vi "one - Server.vi"() -> ()   [LabVIEW 2015]
doc: "This is the TCP server VI that supports multiple connections from client VIs."
uses:
  TCP Multiple Connections/controls/TCP Multiple Connections State.ctl
  TCP Multiple Connections/controls/TCP Multiple Connections Data.ctl
  <vilib>/myRIO/Instrument Drivers/Onboard IO/AI/typedefs/AI Reference.ctl
  <vilib>/myRIO/Common/Instrument Driver Framework/Utilities/typedefs/myRIO Generic Hardware Reference.ctl
  <vilib>/myRIO/Common/Instrument Driver Framework/Utilities/typedefs/Hardware Version Enum.ctl
  <vilib>/myRIO/Common/Instrument Driver Framework/Utilities/typedefs/myRIO v1.0 Reference.ctl
  <vilib>/myRIO/Common/Instrument Driver Framework/Utilities/typedefs/Generic FPGA Reference.ctl
  <vilib>/myRIO/Common/Instrument Driver Framework/myRIO v1.0/AI/typedefs/AI Channels List.ctl
  <vilib>/myRIO/Common/Instrument Driver Framework/myRIO v1.0/AI/typedefs/AI Channels Enum.ctl
  <vilib>/myRIO/Common/Instrument Driver Framework/Utilities/typedefs/Analog Scaling Constants List.ctl
  <vilib>/myRIO/Common/Instrument Driver Framework/Utilities/typedefs/Analog Scaling Constants.ctl
  <vilib>/userdefined/High Color/nirio_resource_hc.ctl
  <vilib>/myRIO/Common/Instrument Driver Framework/Utilities/vis/Is FPGA Ref Available.vi
  <vilib>/myRIO/Common/Instrument Driver Framework/myRIO v1.0/AI/vis/myRIO v1.1 Open AI.vi
  <vilib>/myRIO/Instrument Drivers/Onboard IO/AI/vis/Read.vi
  <vilib>/myRIO/Common/Instrument Driver Framework/Utilities/vis/Validate Channels.vi
  <vilib>/myRIO/Common/Instrument Driver Framework/myRIO v1.0/AI/vis/myRIO v1.0 Reserve AI.vi
  <vilib>/myRIO/Common/Instrument Driver Framework/myRIO v1.0/AI/vis/myRIO v1.0 Build MUX Configuration AI.vi
  <vilib>/myRIO/Common/Instrument Driver Framework/myRIO v1.0/Resource Manager/vis/myRIO v1.0 Reserve Channel List.vi
  <vilib>/myRIO/Common/Instrument Driver Framework/myRIO v1.0/Resource Manager/vis/myRIO v1.0 Reserve Channel.vi
  <vilib>/myRIO/Common/Instrument Driver Framework/myRIO v1.0/Resource Manager/vis/myRIO v1.0 Unreserve Channel.vi
  <vilib>/myRIO/Common/Instrument Driver Framework/myRIO v1.0/Resource Manager/vis/myRIO v1.0 Build Mutex Name.vi
  <vilib>/Utility/VariantDataType/GetNumericInfo.vi
  <vilib>/Utility/error.llb/Error Cluster From Error Code.vi
  <vilib>/myRIO/Common/Instrument Driver Framework/myRIO v1.0/myRIO v1.1 Open.vi
  <vilib>/myRIO/Common/Instrument Driver Framework/myRIO v1.0/AI/vis/myRIO v1.0 Get Scaling Constants AI.vi
  <vilib>/myRIO/Common/Instrument Driver Framework/Utilities/vis/IO Manager.vi
  <vilib>/myRIO/Common/Instrument Driver Framework/Utilities/vis/Configuration Manager.vi
  <vilib>/myRIO/Common/Instrument Driver Framework/myRIO v1.0/myRIO v1.0 Close.vi
  <vilib>/myRIO/Common/Instrument Driver Framework/myRIO v1.0/AI/vis/myRIO v1.0 Read AI.vi
  <vilib>/myRIO/Express VI/Onboard IO/AI/AI Express VI.xnode
  <vilib>/myRIO/Instrument Drivers/Onboard IO/AI/vis/myRIO AI Open.xnode
  <vilib>/myRIO/Instrument Drivers/Onboard IO/AI/AI.lvlib
panel:
  out "String 6":string
  out "Waveform Chart 5":dbl(graph)
  out "String 5":string
  out "Waveform Chart 4":dbl(graph)
  out "String 4":string
  out "Waveform Chart 3":dbl(graph)
  in  "Stop":bool
  out "# of Connections":i32
  # "Overview: Demonstrates the use of the TCP functions to initialize a TCP server that can send data to multiple client VIs.\nInstructions:\n1. Run the VI.\n2. Open TCP Multiple Connections - Client 1.vi and follow the instructions on its front panel.\n3. Open TCP Multiple Connections - Client 2.vi and follow the instructions on its front panel.\n4. Click Stop to stop the VI."
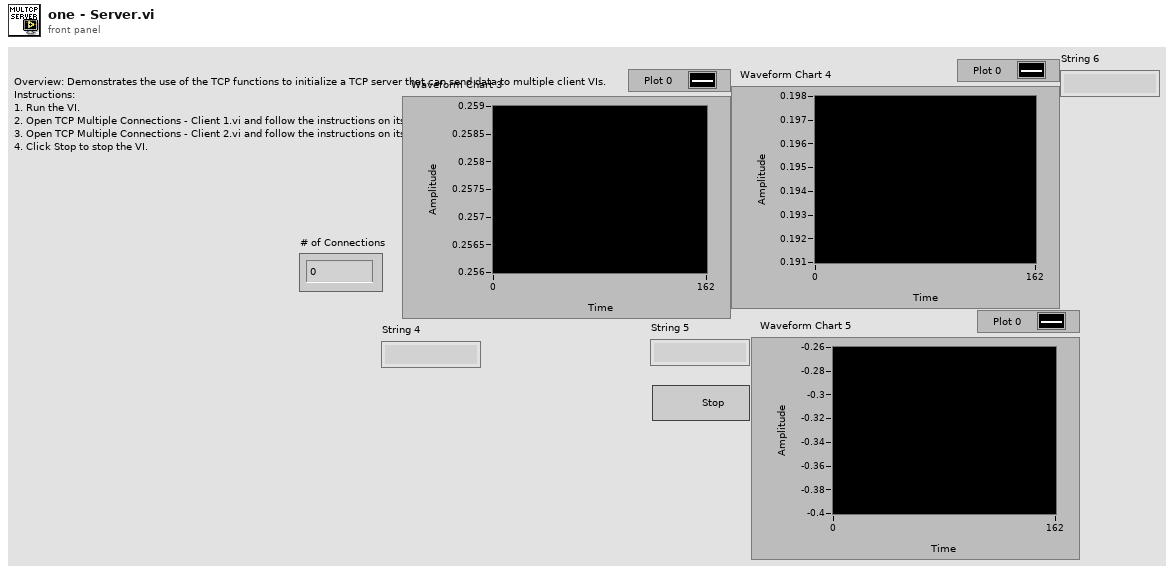
[diagram p1: front panel]
types:
  T1 = typedef "TCP Multiple Connections Data.ctl" = cluster{"Clients":refnum<k5>[], "Listener":refnum<k5>}
  T2 = typedef "TCP Multiple Connections State.ctl" = enum16{"Initialize", "Status Check", "Send Data", "Stop"}
  T3 = typedef "AI.lvlib/AI Reference.ctl" = cluster{"myRIO Reference":T4, "AI Channels List":T8, "AI Scaling Constants List":T10}
  T4 = typedef "myRIO Generic Hardware Reference.ctl" = cluster{"myRIO Model":T5, "myRIO Hardware Reference":T6}
  T5 = typedef "Hardware Version Enum.ctl" = enum16{"Unknown", "myRIO-1900", "myRIO-1950", "roboRIO"}
  T6 = typedef "myRIO v1.0 Reference.ctl" = cluster{"Generic FPGA Reference":T7, "Allow multiple opens":bool}
  T7 = typedef "Generic FPGA Reference.ctl" = refnum<k20>
  T8 = typedef "AI Channels List.ctl" = T9[]
  T9 = typedef "AI Channels Enum.ctl" = enum16{"Not Connected", "AudioIn/Left", "AudioIn/Right", "C/AI0", "C/AI1", "A/AI0", "A/AI1", "A/AI2", "A/AI3", "B/AI0", "B/AI1", "B/AI2", "B/AI3", "AI/AI0", "AI/AI1", "AI/AI2", "AI/AI3"}
  T10 = typedef "Analog Scaling Constants List.ctl" = T11[]
  T11 = typedef "Analog Scaling Constants.ctl" = cluster{"LSB Weight (Volts)":dbl, "Offset (Volts)":dbl, "Signed?":bool}
  T12 = typedef "nirio_resource_hc.ctl" = tag
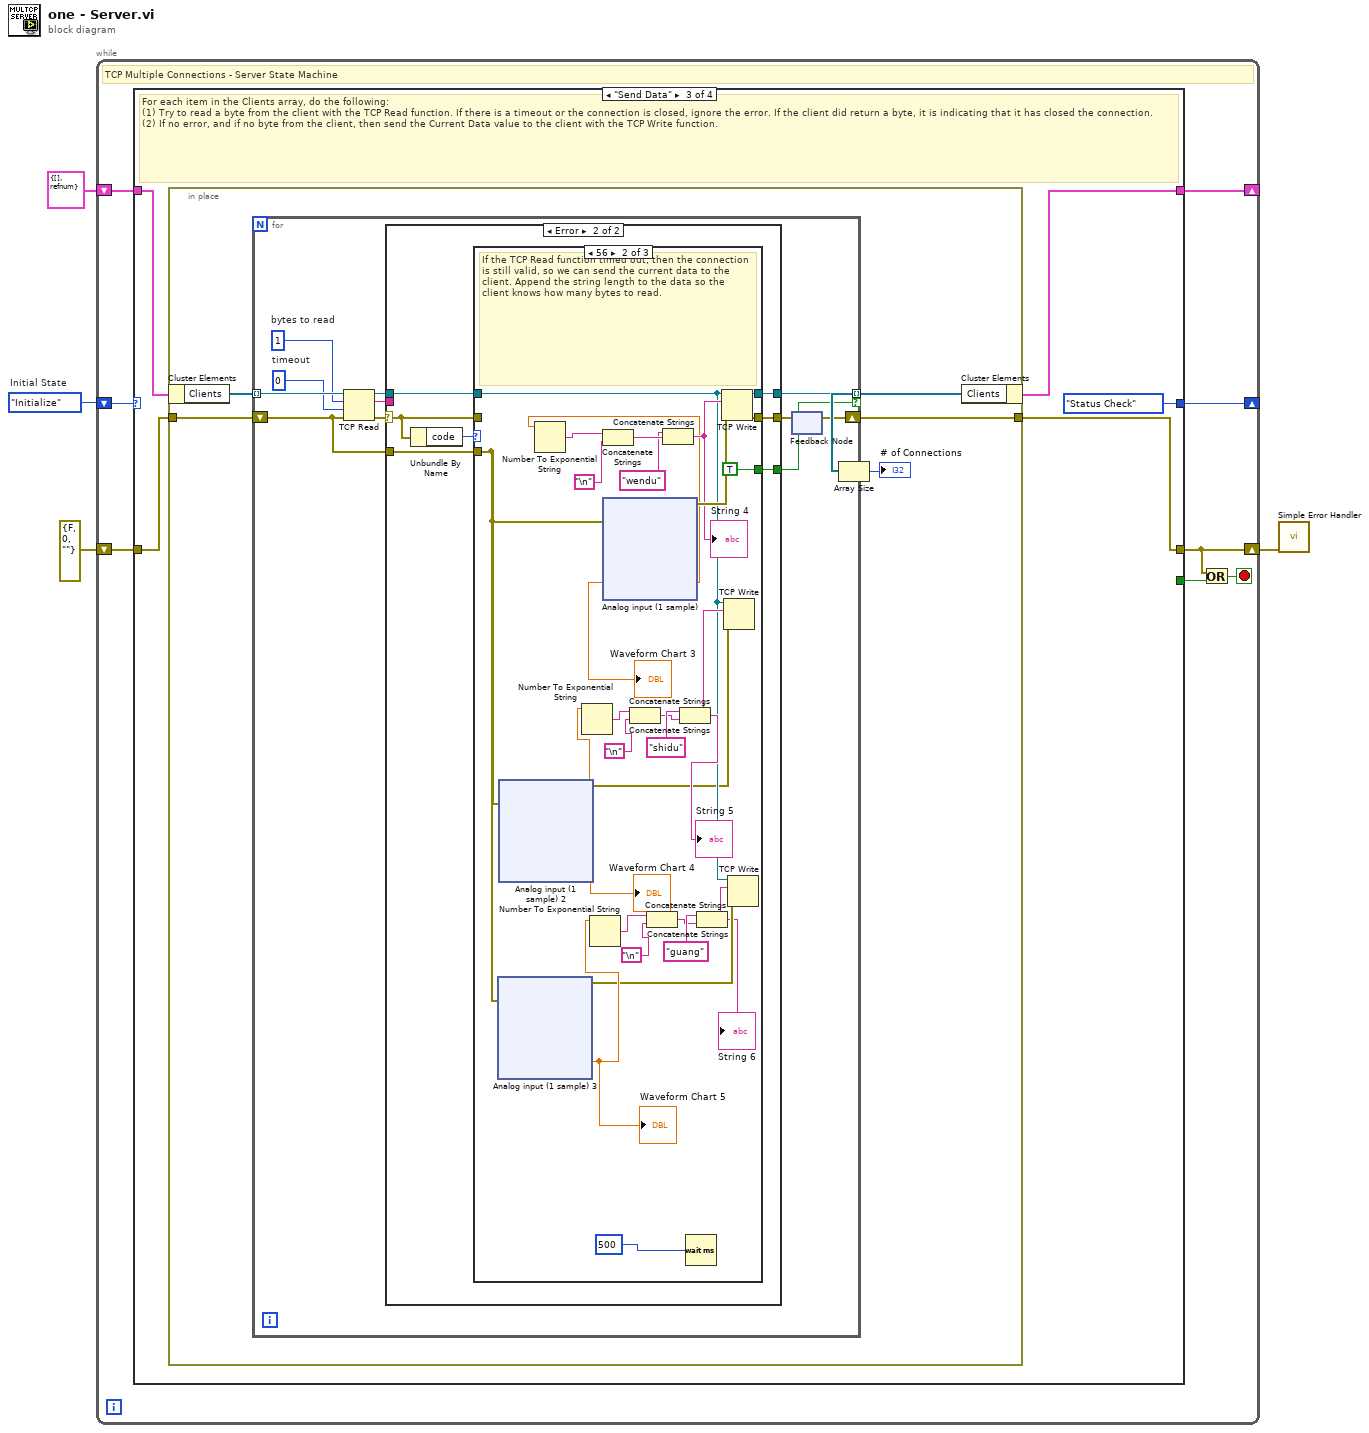
[diagram p0: block diagram]
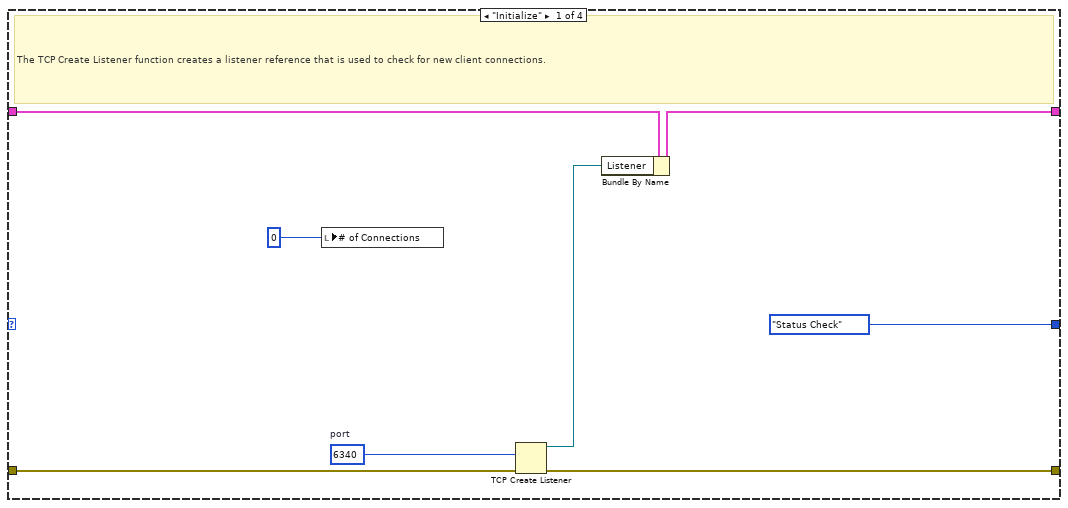
[diagram p2: hidden frame]
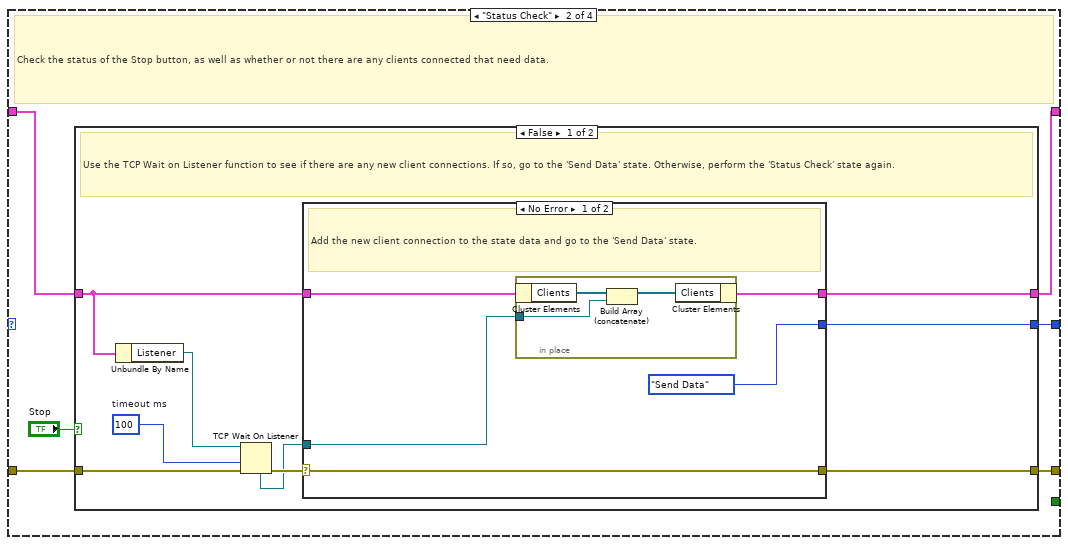
[diagram p3: hidden frame]
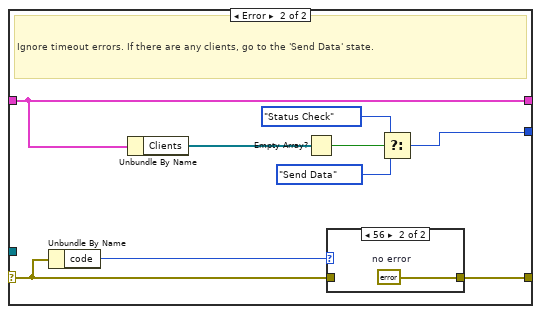
[diagram p4: hidden frame]
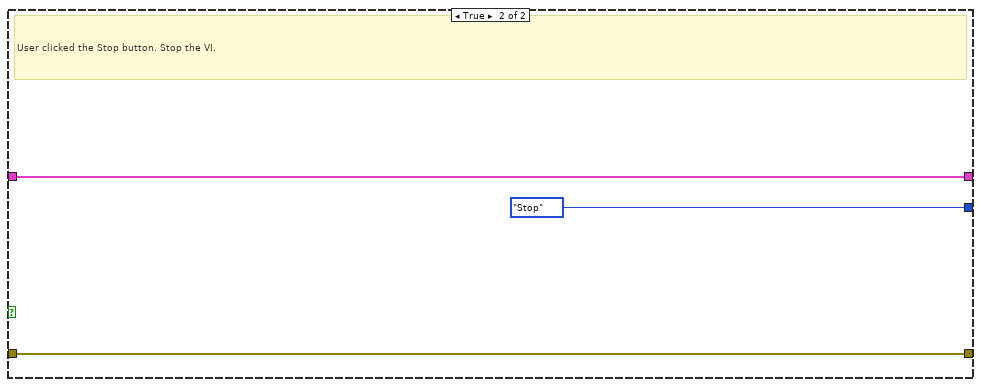
[diagram p6: hidden frame]
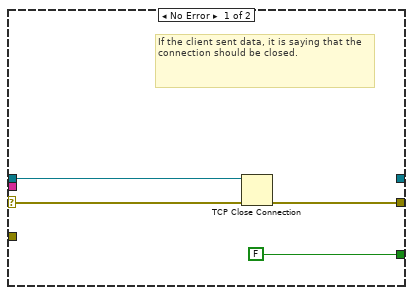
[diagram p7: hidden frame]
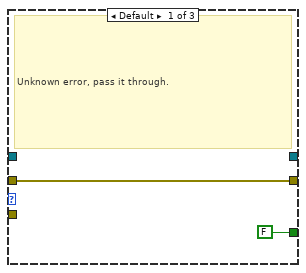
[diagram p8: hidden frame]
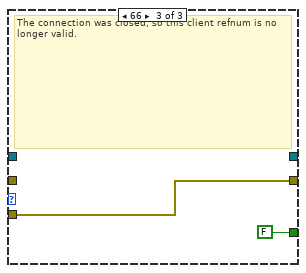
[diagram p9: hidden frame]
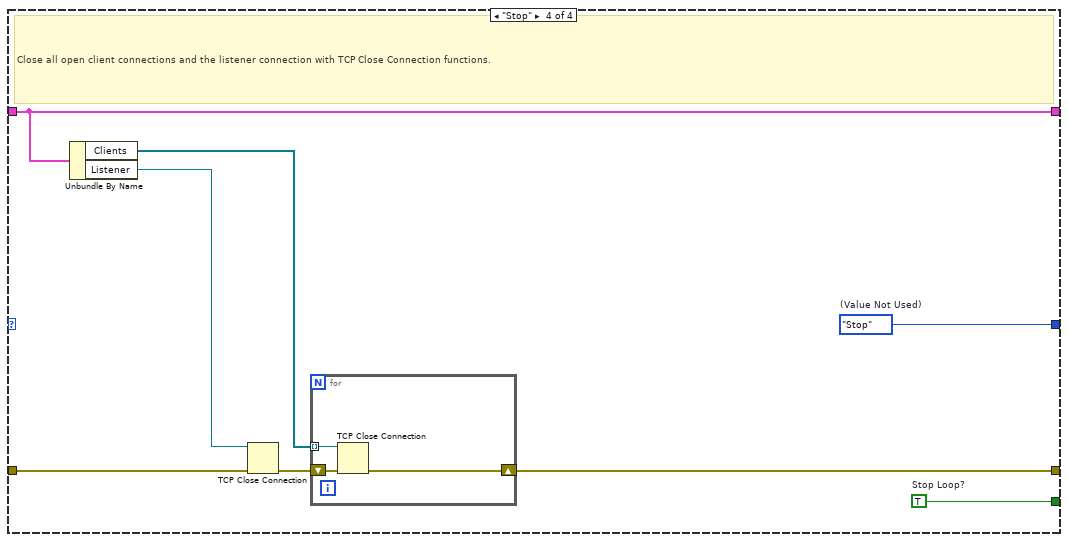
[diagram p10: hidden frame]
diagram:
  w4 = TCP_Multiple_Connections_State."Initialize"  # Initial State
  n1 = while {
    shift-right: [w11] -> _
    shift-left: w4 -> [w12]
    shift-right: [w9] -> _
    shift-left: T1 {"Clients"=[], "Listener"=refnum} ("Data") -> [w10]
    shift-right: [w5] -> w1
    shift-left: errorcluster {"status"=FALSE, "code"=0, "source"=""} ("error constant") -> [w8]
    stop <- w6 stop-if-true
    # "TCP Multiple Connections - Server State Machine"
    n2 = case shown="\"Send Data\"" w12 {
      tunnel: [TCP_Multiple_Connections_State."Status Check" ("States") w26 TCP_Multiple_Connections_State."Status Check" ("States") w232] -> w11
      tunnel: [_ _ _ w239] -> w7
      tunnel: w10 -> [w18 w22 w60 w238]
      tunnel: [w17 w21 w59 w238] -> w9
      tunnel: w8 -> [w20 w25 w62 w237]
      tunnel: [w19 w24 w61 w235] -> w5
      frame "Initialize" {
        w15 = u16 6340  # port
        # "The TCP Create Listener function creates a listener reference that is used to check for new client connections."
        n3 = local write "# of Connections"(0 ("Number of Client Connections")) -> ()
        n4 = TCP Create Listener(8:w20, 10:w15) -> (0:w19:errorcluster, 3:w16:refnum<k5>)  [unwired: 4 out]
        n5 = Bundle By Name(cluster=w18, "Listener"=w16) -> (w17:T1)
      }
      frame "Status Check" {
        # "Check the status of the Stop button, as well as whether or not there are any clients connected that need data."
        n6 = case shown="False" "Stop" {
          tunnel: [w35 TCP_Multiple_Connections_State."Stop" ("States")] -> w26
          tunnel: w25 -> [w34 w57]
          tunnel: [w27 w57] -> w24
          tunnel: w22 -> [w30 w56]
          tunnel: [w29 w56] -> w21
          frame False {
            w33 = 100  # timeout ms
            # "Use the TCP Wait on Listener function to see if there are any new client connections. If so, go to the 'Send Data' state. Otherwise, perform the 'Status Check' state again."
            n7 = Unbundle By Name(w30) -> ("Listener"=w28:refnum<k5>)
            n8 = TCP Wait On Listener(8:w34, 9:w33, 11:w28) -> (0:w32:errorcluster, 4:w31:refnum<k5>)  [unwired: 4 out]
            n9 = case shown="No Error" w32 {
              selector: w32 -> [w38 w52]
              tunnel: [TCP_Multiple_Connections_State."Send Data" ("States") w46] -> w35
              tunnel: w31 -> [w39 _]
              tunnel: w30 -> [w40 w49]
              tunnel: [w37 w49] -> w29
              tunnel: [w38 w50] -> w27
              frame No Error {
                # "Add the new client connection to the state data and go to the 'Send Data' state."
                n10 = in-place {
                  in-place-border: w39 -> [w41]
                  n11 = in-place-cluster #1(w40) -> ("Clients"=w43:refnum<k5>[])
                  n12 = Build Array (concatenate)(w43, w41) -> (w42:refnum<k5>[])
                  n13 = in-place-cluster #1("Clients"=w42) -> (w37:T1)
                }
              }
              frame Error {
                # "Ignore timeout errors. If there are any clients, go to the 'Send Data' state."
                n14 = Unbundle By Name(w52) -> ("code"=w51:i32)
                n15 = Unbundle By Name(w49) -> ("Clients"=w48:refnum<k5>[])
                n16 = Empty Array?(array=w48) -> (empty?=w47:bool)
                n17 = case shown="56" w51 {
                  tunnel: w52 -> [w53 _]
                  tunnel: [w53 w54] -> w50
                  frame Default {
                  }
                  frame 56 {
                    w54 = errorcluster {"status"=FALSE, "code"=0, "source"=""}  # no error
                  }
                }
                n18 = Select(t=TCP_Multiple_Connections_State."Status Check" ("States"), s=w47, f=TCP_Multiple_Connections_State."Send Data" ("States")) -> (s? t:f=w46:T2)
              }
            }
          }
          frame True {
            # "User clicked the Stop button. Stop the VI."
          }
        }
      }
      frame "Send Data" {
        # "For each item in the Clients array, do the following:\n(1) Try to read a byte from the client with the TCP Read function. If there is a timeout or the connection is closed, ignore the error. If the client did return a byte, it is indicating that it has closed the connection.\n(2) If no error, and if no byte from the client, then send the Current Data value to the client with the TCP Write function."
        n19 = in-place {
          in-place-border: w62 -> [w67]
          in-place-border: [w66] -> w61
          n20 = in-place-cluster #2(w60) -> ("Clients"=w64:refnum<k5>[])
          n21 = for {
            tunnel: w64 -> [w78] mode=indexing
            shift-right: [w68] -> w66
            shift-left: w67 -> [w70]
            tunnel: [w72] -> w63 mode=indexing if=w71
            w75 = 0  # timeout
            w76 = 1  # bytes to read
            n22 = TCP Read(connection ID=w78, bytes to read=w76, error in (no error)=w70, 9:w75) -> (connection ID out=w77:refnum<k5>, data out=w73:string, error out=w74:errorcluster)  [unwired: 1 out]
            n23 = case shown="Error" w74 {
              selector: w74 -> [w81 w88]
              tunnel: w77 -> [w82 w85]
              tunnel: w73 -> [_ _]
              tunnel: [_ w83] -> w72
              tunnel: [FALSE w84] -> w71
              tunnel: [w79 w87] -> w69
              tunnel: w70 -> [_ w86]
              frame No Error {
                # "If the client sent data, it is saying that the connection should be closed."
                # "If the client sent data, it is saying that the connection should be closed."
                n24 = TCP Close Connection(connection ID=w82, error in (no error)=w81) -> (error out=w79:errorcluster)  [unwired: 2 out]
              }
              frame Error {
                # "Ignore connection closed and timeout errors"
                n25 = Unbundle By Name(w88) -> ("code"=w89:i32)
                n26 = case shown="56" w89 {
                  tunnel: w88 -> [w91 _ _]
                  tunnel: [w91 w118 w231] -> w87
                  tunnel: w86 -> [_ w97 w231]
                  tunnel: w85 -> [_ w101 _]
                  tunnel: [FALSE TRUE FALSE] -> w84
                  tunnel: [_ w117 _] -> w83
                  frame Default {
                    # "Unknown error, pass it through."
                  }
                  frame 56 {
                    # "If the TCP Read function timed out, then the connection is still valid, so we can send the current data to the client. Append the string length to the data so the client knows how many bytes to read."
                    n27 = xnode "Analog input (1 sample) 3"("error in (no error)"=w97) -> ("C/AI0 (AI0)"=w104:dbl, "error out"=w100:errorcluster)
                    "Waveform Chart 5" <- w104
                    n28 = xnode "Analog input (1 sample) 2"("error in (no error)"=w97) -> ("B/AI0 (Pin 3)"=w99:dbl, "error out"=w98:errorcluster)
                    "Waveform Chart 4" <- w99
                    n29 = Number To Exponential String(number=w99) -> (E-format string=w107:string)  [unwired: 3 in]
                    n30 = Number To Exponential String(number=w104) -> (E-format string=w102:string)  [unwired: 3 in]
                    n31 = xnode "Analog input (1 sample)"("error in (no error)"=w97) -> ("A/AI0 (Pin 3)"=w109:dbl, "error out"=w115:errorcluster)
                    "Waveform Chart 3" <- w109
                    n32 = Number To Exponential String(number=w109) -> (E-format string=w111:string)  [unwired: 3 in]
                    n33 = Concatenate Strings(w111, "\n") -> (w113:string)
                    n34 = Concatenate Strings(w107, "\n") -> (w93:string)
                    n35 = Concatenate Strings(w102, "\n") -> (w95:string)
                    n36 = Concatenate Strings("wendu", w113) -> (w110:string)
                    "String 4" <- w110
                    n37 = Concatenate Strings("shidu", w93) -> (w105:string)
                    "String 5" <- w105
                    n38 = Wait (ms)(milliseconds to wait=500) -> ()  [unwired: 1 out]
                    n39 = Concatenate Strings("guang", w95) -> (w92:string)
                    "String 6" <- w92
                    n40 = TCP Write(connection ID=w101, data in=w110, error in (no error)=w115) -> (connection ID out=w117:refnum<k5>, error out=w118:errorcluster)  [unwired: 2 out]
                    n41 = TCP Write(connection ID=w101, data in=w105, error in (no error)=w98) -> ()  [unwired: 1 in, 3 out]
                    n42 = TCP Write(connection ID=w101, data in=w92, error in (no error)=w100) -> ()  [unwired: 1 in, 3 out]
                  }
                  frame 66 {
                    # "The connection was closed, so this client refnum is no longer valid."
                  }
                }
              }
            }
            n43 = feedback-in #3(w69) -> ()
            n44 = feedback #3() -> (w68:errorcluster)  [unwired: 1 in]
          }
          n45 = Array Size(array=w63) -> (size(s)=→"# of Connections":i32)
          n46 = in-place-cluster #2("Clients"=w63) -> (w59:T1)
        }
      }
      frame "Stop" {
        w232 = TCP_Multiple_Connections_State."Stop"  # (Value Not Used)
        w239 = TRUE  # Stop Loop?
        # "Close all open client connections and the listener connection with TCP Close Connection functions."
        n47 = Unbundle By Name(w238) -> ("Clients"=w236:refnum<k5>[], "Listener"=w233:refnum<k5>)
        n48 = TCP Close Connection(connection ID=w233, error in (no error)=w237) -> (error out=w234:errorcluster)  [unwired: 1 in, 1 out]
        n49 = for {
          shift-right: [w241] -> w235
          shift-left: w234 -> [w242]
          tunnel: w236 -> [w240] mode=indexing
          n50 = TCP Close Connection(connection ID=w240, error in (no error)=w242) -> (error out=w241:errorcluster)  [unwired: 1 in, 1 out]
        }
      }
    }
    n51 = Or(x=w5, y=w7) -> (x .or. y?=w6:bool)
  }
  n52 = call <vilib>:"Simple Error Handler.vi"("error in (no error)"=w1) -> ()  [unwired: 4 in, 5 out]
